vi "AutoScaleTime (SubVI).vi"(9 "Numeric 3":i32, 10 "TblPrm2":sgl[][](array[numeric]), 11 "TableParam 0":sgl[][](array[numeric])) -> (2 "Numeric 2":sgl, 3 "Numeric":sgl)   [LabVIEW 2017]
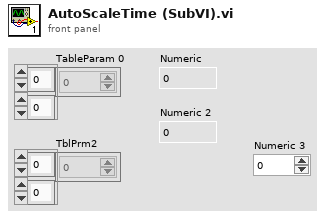
[diagram p1: front panel]
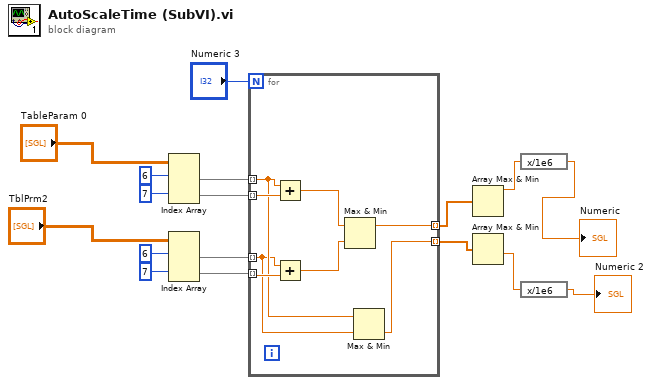
[diagram p0: block diagram]
diagram:
  n1 = Index Array(array="TableParam 0", index (row) #1=6 ("index (row)"), index (row) #2=7 ("disabled index (col)")) -> (element #1=w12:sgl[], element #2=w13:sgl[])  [unwired: 2 in]
  n2 = Index Array(array="TblPrm2", index (row) #1=6 ("index (row)"), index (row) #2=7 ("disabled index (col)")) -> (element #1=w14:sgl[], element #2=w15:sgl[])  [unwired: 2 in]
  n3 = for {
    N: "Numeric 3" -> [_]
    tunnel: w12 -> [w20] mode=indexing
    tunnel: w13 -> [w25] mode=indexing
    tunnel: w14 -> [w19] mode=indexing
    tunnel: w15 -> [w24] mode=indexing
    tunnel: [w21] -> w16 mode=indexing
    tunnel: [w18] -> w17 mode=indexing
    n4 = Add(x=w20, y=w25) -> (x+y=w23:sgl)
    n5 = Add(x=w19, y=w24) -> (x+y=w22:sgl)
    n6 = Max & Min(x=w23, y=w22) -> (max(x,y)=w21:sgl)  [unwired: 1 out]
    n7 = Max & Min(x=w20, y=w19) -> (min(x,y)=w18:sgl)  [unwired: 1 out]
  }
  n8 = Array Max & Min(array=w16) -> (max value=w3:sgl)  [unwired: 3 out]
  n9 = Array Max & Min(array=w17) -> (min value=w5:sgl)  [unwired: 3 out]
  n10 = expression code="x/1e6"(w3) -> (→"Numeric":sgl)
  n11 = expression code="x/1e6"(w5) -> (→"Numeric 2":sgl)
